vi "Save Configuration Settings to XML.vi"(8 "error in (no error)":errorcluster, 11 "User Configuration":T1={"Hardware Configuration"={"VGC50"={"serial settings"={"port"="", "baud rate"=115200}, "device information"={"type"="", "model number"="", "serial number"="", "firmware version"="", "hardware version"=""}, "VGC"=refnum, "Backing SP"={"mode"=0, "thresholds"={"lower"=0.0, "upper"=0.0}, "on"=FALSE}, "Chamber SP"={"mode"=1, "thresholds"={"lower"=0.0, "upper"=0.0}, "on"=FALSE}}, "PTC10"={"serial settings"={"port"="GPIB0::22::INSTR", "baud rate"=115200}, "PTC10 Info"={"Manufacturer"="", "Instrument"="", "Serial Number"="", "Firmware"=""}, "VISA resource name"="", "pwmloop"="define pwmloop(#t=0 while (1) {waitforsample if(#pwm=0){relays=0}else{if(#t<#pwm) {relays=1}else{relays=3}}#t+=1 if  (#t>99){#t=0} pause 0.2 s})", "onecycle"="define onecycle (pwm=100 run pwmloop 5A.PID.Setpoint=-130.0 5A.PID.input=3C while(#3C>-129.0){pause 0.2 s}pwm=-130 pause 10 min pwm=0  5A.PID.SetPoint=50.0 while(#3C<49.0){pause 0.2 s} pause 10 min kill pwmloop)", "control"="define control (#count=1 while (#count>=0) {onecycle pause 1 s #count-=1})", "HeatDrive"="define Failsafe (while(1) {if (#Check <-20){relays=0 outputEnable Off}else{if(#Check>20){relays=0 outputEnable Off}} pause 1 s})", "ToAmbient"="define ToAmbient(if(#3C>25.0){pwm=100 run pwmloop while(#3C>#25.0){pause 0.5 s} pwm=0 kill pwmloop}else{#5A.PID.setpoint=20.0 while(#3C<15.0){pause 0.5 s} outputenable off})", "StartupCode"="system.display.Monitors Show", "LogChannels"=[], "Heater O/P Channel"="", " Control Input"="", "TAmbient"=20.0, "AmbientTolerance"=5.0, "TestCycleParameters"={"TAmb"=20.0, "HeaterTestTemp"=51.5, "HeaterTestDwell(min)"=20, "HeaterTestDuration"=20, "MinOpTemp"=1.0, "MinOpDwell(min)"=1, "TestHeatingRate (deg/min)"=-131.5, "SurviveCycleParameters"={"MinSurviveTemp"=-131.5, "MinSurvive Dwell(min)"=10, "MaxSurviveTemp"=50.0, "MaxSurviveDwell(min)"=30, "ControlInput"=2, "ColdStandOff"=4.0, "HotStandoff"=5.0, "SteadyPWM"=20, "MaxCoolingRate (deg/min)"=3.75, "MaxHeatingRate (deg/min)"=2.5}, "CycleType"=0, "MaxOpTemp"=-50.0, "MaxOpDwell(min)"=30}, "PID Params"={"P"=1.14, "I"=0.012, "D"=21.68, "Set"=0.0}}}, "Vacuum Graph config"={"Log/Lin"=FALSE, "Show Backing"=FALSE, "Show Chamber"=FALSE}} {"Hardware Configuration"."PTC10"."PID Params"."D" min=0.0; "Hardware Configuration"."PTC10"."PID Params"."I" min=0.0; "Hardware Configuration"."PTC10"."PID Params"."P" min=0.0; "Hardware Configuration"."PTC10"."TestCycleParameters"."CycleType" items=["Survival", "Operational"]; "Hardware Configuration"."PTC10"."TestCycleParameters"."SurviveCycleParameters"."SteadyPWM" min=0 max=100 step=1; "Hardware Configuration"."PTC10"."TestCycleParameters"."SurviveCycleParameters"."ControlInput" items=["3A", "3B", "3C", "3D", "4A", "4B", "4C", "4D"]; "Hardware Configuration"."PTC10"."serial settings"."baud rate" items=["9600"=9600, "19200"=19200, "38400"=38400, "57600"=57600, "115200"=115200]; "Hardware Configuration"."VGC50"."Chamber SP"."thresholds"."upper" format="%#_5p"; "Hardware Configuration"."VGC50"."Chamber SP"."thresholds"."lower" format="%#_5p"; "Hardware Configuration"."VGC50"."Chamber SP"."mode" items=["off", "on", "channel 1", "channel 2", "channel 3"]; "Hardware Configuration"."VGC50"."Backing SP"."thresholds"."upper" format="%#_5p"; "Hardware Configuration"."VGC50"."Backing SP"."thresholds"."lower" format="%#_5p"; "Hardware Configuration"."VGC50"."Backing SP"."mode" items=["off", "on", "channel 1", "channel 2", "channel 3"]; "Hardware Configuration"."VGC50"."serial settings"."baud rate" items=["9600"=9600, "19200"=19200, "38400"=38400, "57600"=57600, "115200"=115200]}) -> (0 "error out":errorcluster)   [LabVIEW 2024]
doc: "Saves the user-specified configuration data to an XML file. This is used to remember settings between executions."
uses:
  controls/User Specified Data.ctl
  <instrlib>/PL Inficon VGC/PL Inficon VGC.lvclass
  controls/HW Configuration.ctl
  controls/VGC50.ctl
  controls/SRS PTC10.ctl
  controls/TestCycleParams.ctl
  controls/SurviveCycleParams.ctl
  controls/ControlInput.ctl
  controls/PID Params.ctl
  controls/Vac Graph Config.ctl
  <vilib>/Utility/xml.llb/Write to XML File(string).vi
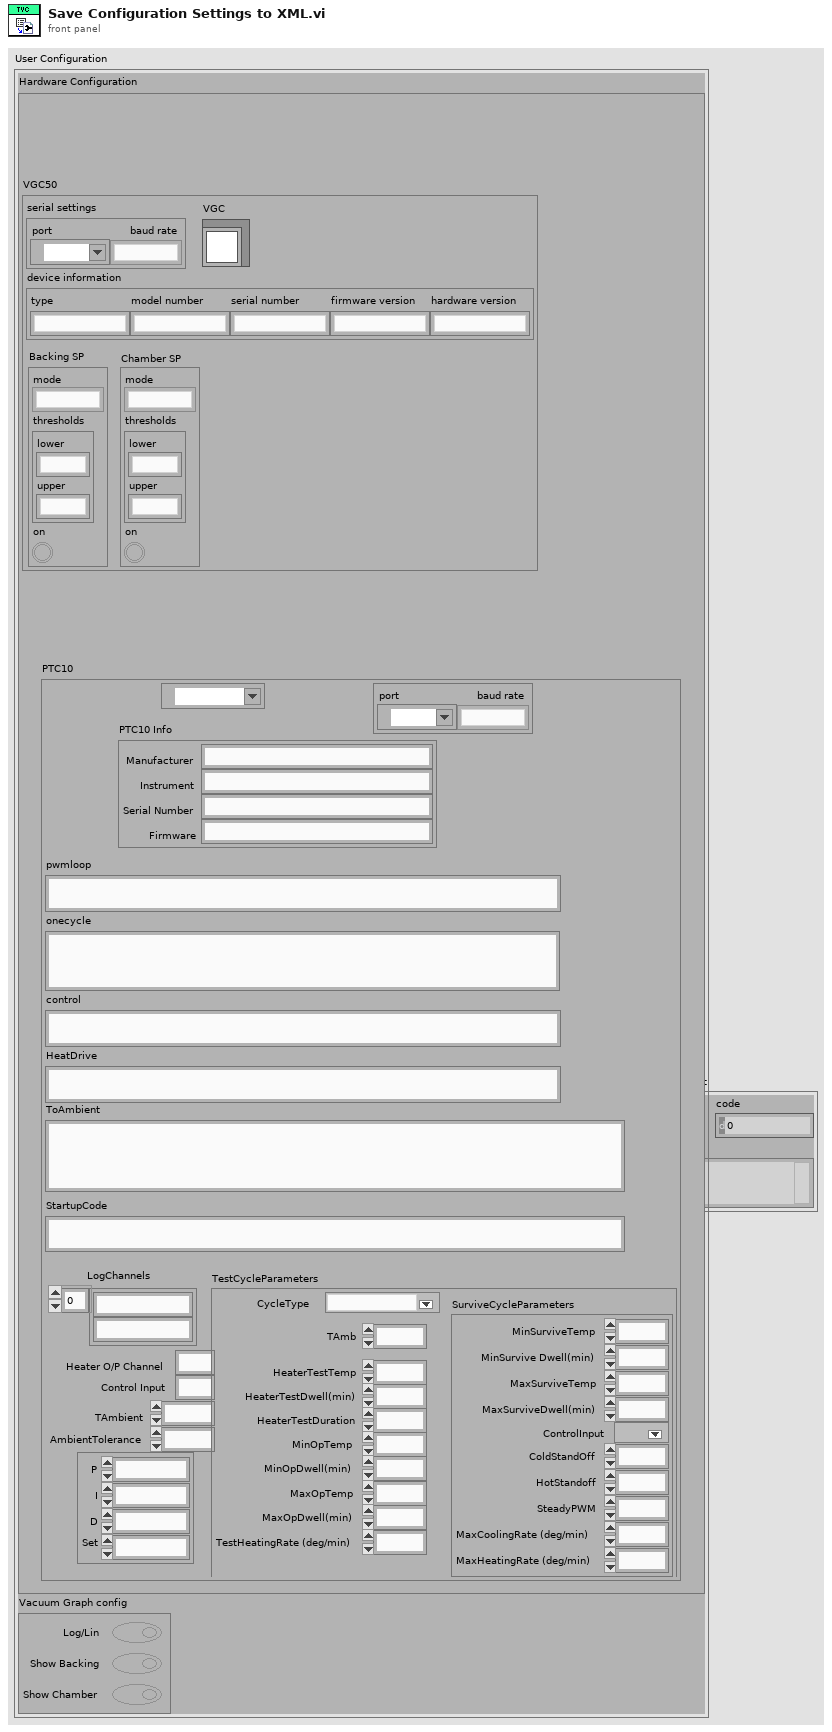
[diagram p1: front panel]
types:
  T1 = typedef "User Specified Data.ctl" = cluster{"Hardware Configuration":T2, "Vacuum Graph config":T9}
  T2 = typedef "HW Configuration.ctl" = cluster{"VGC50":T3, "PTC10":T4}
  T3 = typedef "VGC50.ctl" = cluster{"serial settings":cluster{"port":refnum<visa-resource-name>, "baud rate":u32}, "device information":cluster{"type":string, "model number":string, "serial number":string, "firmware version":string, "hardware version":string}, "VGC":refnum<class "PL Inficon VGC.lvclass">, "Backing SP":cluster{"mode":u16, "thresholds":cluster{"lower":dbl, "upper":dbl}, "on":bool}, "Chamber SP":cluster{"mode":u16, "thresholds":cluster{"lower":dbl, "upper":dbl}, "on":bool}}
  T4 = typedef "SRS PTC10.ctl" = cluster{"serial settings":cluster{"port":refnum<visa-resource-name>, "baud rate":u32}, "PTC10 Info":cluster{"Manufacturer":string, "Instrument":string, "Serial Number":string, "Firmware":string}, "VISA resource name":refnum<visa-resource-name>, "pwmloop":string, "onecycle":string, "control":string, "HeatDrive":string, "ToAmbient":string, "StartupCode":string, "LogChannels":string[], "Heater O/P Channel":string, " Control Input":string, "TAmbient":dbl, "AmbientTolerance":dbl, "TestCycleParameters":T5, "PID Params":T8}
  T5 = typedef "TestCycleParams.ctl" = cluster{"TAmb":dbl, "HeaterTestTemp":dbl, "HeaterTestDwell(min)":i32, "HeaterTestDuration":i32, "MinOpTemp":dbl, "MinOpDwell(min)":i32, "TestHeatingRate (deg/min)":dbl, "SurviveCycleParameters":T6, "CycleType":u16, "MaxOpTemp":dbl, "MaxOpDwell(min)":i32}
  T6 = typedef "SurviveCycleParams.ctl" = cluster{"MinSurviveTemp":dbl, "MinSurvive Dwell(min)":i32, "MaxSurviveTemp":dbl, "MaxSurviveDwell(min)":i32, "ControlInput":T7, "ColdStandOff":dbl, "HotStandoff":dbl, "SteadyPWM":i32, "MaxCoolingRate (deg/min)":dbl, "MaxHeatingRate (deg/min)":dbl}
  T7 = typedef "ControlInput.ctl" = u16
  T8 = typedef "PID Params.ctl" = cluster{"P":dbl, "I":dbl, "D":dbl, "Set":dbl}
  T9 = typedef "Vac Graph Config.ctl" = cluster{"Log/Lin":bool, "Show Backing":bool, "Show Chamber":bool}
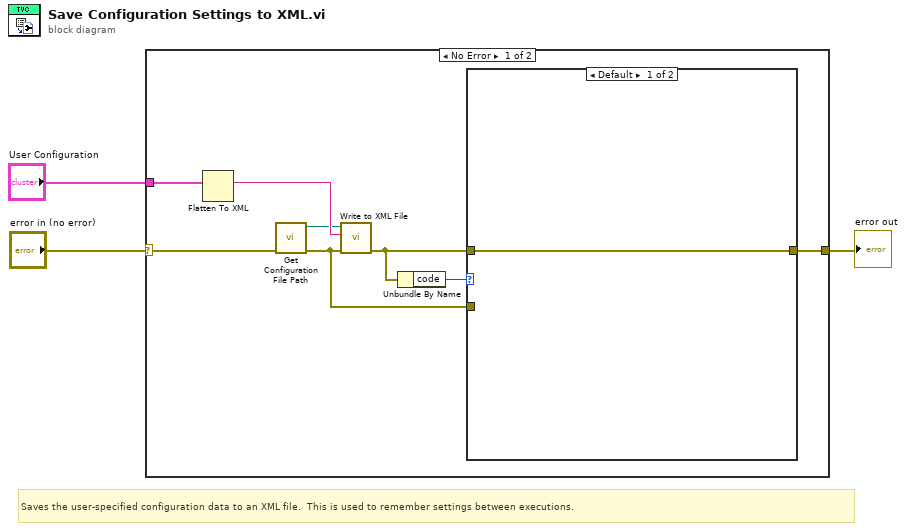
[diagram p0: block diagram]
diagram:
  # "Saves the user-specified configuration data to an XML file.  This is used to remember settings between executions."
  n1 = case shown="No Error" "error in (no error)" {
    selector: "error in (no error)" -> [w8 w14]
    tunnel: [w5 w14] -> w2
    tunnel: "User Configuration" -> [w11 _]
    frame No Error {
      n2 = Flatten To XML(6:w11) -> (2:w10:string)
      n3 = call "Get Configuration File Path.vi"("error in (no error)"=w8) -> ("error out"=w4:errorcluster, "XML File Path"=w9:path)  [unwired: 9 in]
      n4 = call-poly <vilib>:"Write to XML File.vi"("error in (no error)"=w4, "XML Input"=w10, "XML File Path"=w9) -> ("error out"=w6:errorcluster)  [unwired: 6 in, 2 out]
      n5 = Unbundle By Name(w6) -> ("code"=w7:i32)
      n6 = case shown="Default" w7 {
        tunnel: [w12 w13] -> w5
        tunnel: w6 -> [w12 _]
        tunnel: w4 -> [_ w13]
        frame Default {
        }
        frame 8 {
          # "Ignore a permissions error when attempting to save the Settings.xml file."
          # "#CodeRecommended - Add code here to perform additional actions if a permissions error occurs when saving the Settings.xml file."
        }
      }
    }
    frame Error {
    }
  }
  "error out" <- w2
